vi "Graph properties.vi"(8 "error in (no error)":errorcluster, 11 "Mixed Signal Graph 3":refnum<vi>) -> (0 "error out":errorcluster)   [LabVIEW 2014]
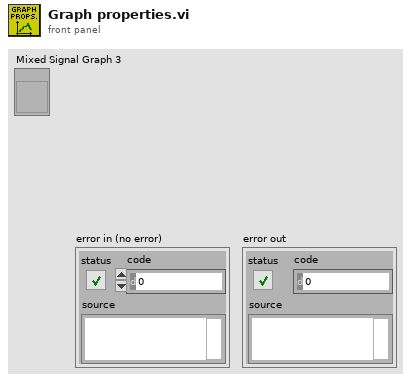
[diagram p1: front panel]
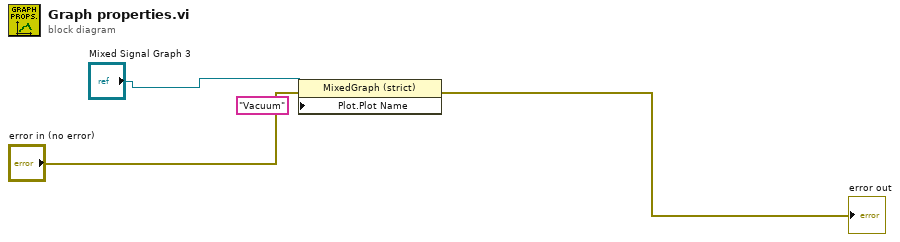
[diagram p0: block diagram]
diagram:
  (unwired) "Vacuum" ("Plot.Plot Name")
  n1 = property class="MixedGraph (strict)" props=["Plot", "Plot Name"](reference="Mixed Signal Graph 3", error in="error in (no error)") -> (error out=→"error out":errorcluster)  [unwired: 1 in, 1 out]
